vi "Get Project Symbols.vi"(6 "Debug Build?":bool, 8 "error in (no error)":errorcluster, 10 "Build Config in":T1, 11 "Refnum in":T2) -> (0 "error out":errorcluster, 2 "Build Config out":T1, 3 "Refnum out":T2)   [LabVIEW 2019, in "PPL INI Parsing.lvlib"]
uses:
  PPL INI Parsing.lvlib
  Build Configuration.ctl
  <vilib>/Utility/config.llb/Config Data RefNum.ctl
  <vilib>/Utility/config.llb/Read Key (String).vi
  <vilib>/Utility/config.llb/NI_LVConfig.lvlib
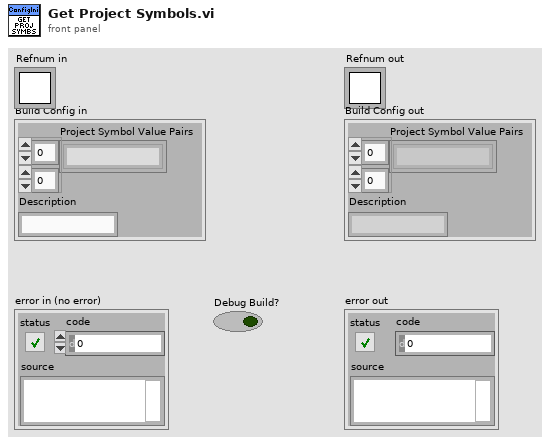
[diagram p1: front panel]
types:
  T1 = typedef "PPL INI Parsing.lvlib/Build Configuration.ctl" = cluster{"SV Pairs":string[][], "Description":string}
  T2 = typedef "NI_LVConfig.lvlib/Config Data RefNum.ctl" = refnum<k1>
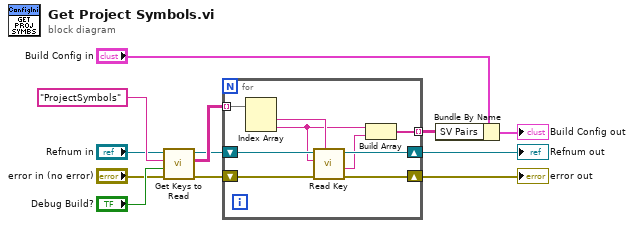
[diagram p0: block diagram]
diagram:
  n1 = call "Get Keys to Read.vi"("error in (no error)"="error in (no error)", "Debug Build?"="Debug Build?", "Section Name"="ProjectSymbols", "Config File"="Refnum in") -> ("error out"=w7:errorcluster, "Keys to Read"=w10:string[][], "Config File"=w5:T2)  [unwired: 5 in]
  n2 = for {
    shift-right: [w19] -> w2
    shift-left: w5 -> [w20]
    shift-right: [w18] -> w3
    shift-left: w7 -> [w21]
    tunnel: w10 -> [w15] mode=indexing
    tunnel: [w16] -> w12 mode=indexing
    n3 = Index Array(array=w15) -> (element #1=w14:string, element #2=w13:string)  [unwired: 2 in]
    n4 = call-poly <vilib>:"Read Key.vi"("section"=w14, "error in (no error)"=w21, "key"=w13, "refnum"=w20) -> ("error out"=w18:errorcluster, "value"=w17:string, "refnum out"=w19:T2)  [unwired: 4 in, 1 out]
    n5 = Build Array(w13, w17) -> (w16:string[])
  }
  "error out" <- w3
  "Refnum out" <- w2
  n6 = Bundle By Name(cluster="Build Config in", "SV Pairs"=w12) -> (→"Build Config out":T1)
